vi "jigglePlatform.vi"(6 "mazeDirection":string, 9 "up or down":string, 11 "Platforms\nto jiggle":dbl[](array[numeric])) -> ()   [LabVIEW 2017]
uses:
  <vilib>/imath/engines/lvmath2/RunTimeEngine/BuiltInFunctions/length/NIMS_length(GV).vi
  <instcachedir>/0/NIMS_length(GV)_08A3D13377FD4E4B96F5795FBF3698FA.lvgen/NIMS_length(GV)_08A3D13377FD4E4B96F5795FBF3698FA_003.vi
  <vilib>/imath/engines/lvmath2/RunTimeEngine/BuiltInFunctions/repeatmx/NIMS_repeatmx(GM, I32, I32).vi
  <instcachedir>/0/NIMS_repeatmx(GM, I32, I32)_8EDBB852F26742A48D04758F158AC943.lvgen/NIMS_repeatmx(GM, I32, I32)_8EDBB852F26742A48D04758F158AC943_004.vi
  <vilib>/imath/engines/lvmath2/RunTimeEngine/RowToken/NIMS_RowToken_SorRV_M.vi
  <instcachedir>/0/NIMS_RowToken_SorRV_M_997882E9B890466D9AE38E5C4E8B9D70.lvgen/NIMS_RowToken_SorRV_M_997882E9B890466D9AE38E5C4E8B9D70_000.vi
  <vilib>/imath/engines/lvmath2/RunTimeEngine/ErrorHandling/NIMS_Create Error From Enums.vi
  <vilib>/imath/engines/lvmath2/RunTimeEngine/BuiltInFunctions/mirrorh/NIMS_mirrorh(GRowV).vi
  <instcachedir>/0/NIMS_mirrorh(GRowV)_B6A8CC4EAFBA4F9A82A59460D67BDFF0.lvgen/NIMS_mirrorh(GRowV)_B6A8CC4EAFBA4F9A82A59460D67BDFF0_000.vi
  <vilib>/imath/engines/lvmath2/RunTimeEngine/MatrixToken/NIMS_MatrixToken_RV_RV.vi
  <instcachedir>/0/NIMS_MatrixToken_RV_RV_8B087EE0EE16477EBE1C341EABB504F3.lvgen/NIMS_MatrixToken_RV_RV_8B087EE0EE16477EBE1C341EABB504F3_002.vi
  <vilib>/imathl/engines/lvmath/Functions/Error Handling/Create Error.vi
  <vilib>/imath/engines/lvmath2/RunTimeEngine/IndexRead/NIMS M($).vi
  <instcachedir>/0/NIMS M($)_82D1177398184AFB96A6AFB63C3C3F57.lvgen/NIMS M($)_82D1177398184AFB96A6AFB63C3C3F57_005.vi
  <vilib>/imath/engines/lvmath2/RunTimeEngine/MatrixToken/NIMS_MatrixToken_M_RV.vi
  <instcachedir>/0/NIMS_MatrixToken_M_RV_EE6E048DE0454E429C3E3ED099F2A9DF.lvgen/NIMS_MatrixToken_M_RV_EE6E048DE0454E429C3E3ED099F2A9DF_002.vi
  <vilib>/imath/engines/lvmath2/RunTimeEngine/NodeEndStatement/NIMS_NodeEndStatement_Output.vi
  <instcachedir>/0/NIMS_NodeEndStatement_Output_53EC0D466D134D7ABD903AC30B43404B.lvgen/NIMS_NodeEndStatement_Output_53EC0D466D134D7ABD903AC30B43404B_012.vi
  <vilib>/imath/engines/lvmath2/RunTimeEngine/ErrorHandling/NIMS_Finalize Error.vi
panel:
  out "Digital Waveform Graph 2":digitalwaveform(graph)
  out "Digital Waveform Graph 3":digitalwaveform(graph)
  out "Digital Waveform Graph":digitalwaveform(graph)
  # "Briefly move the platform.\nUsed to move platform up and down in \norder to convince animal to move."
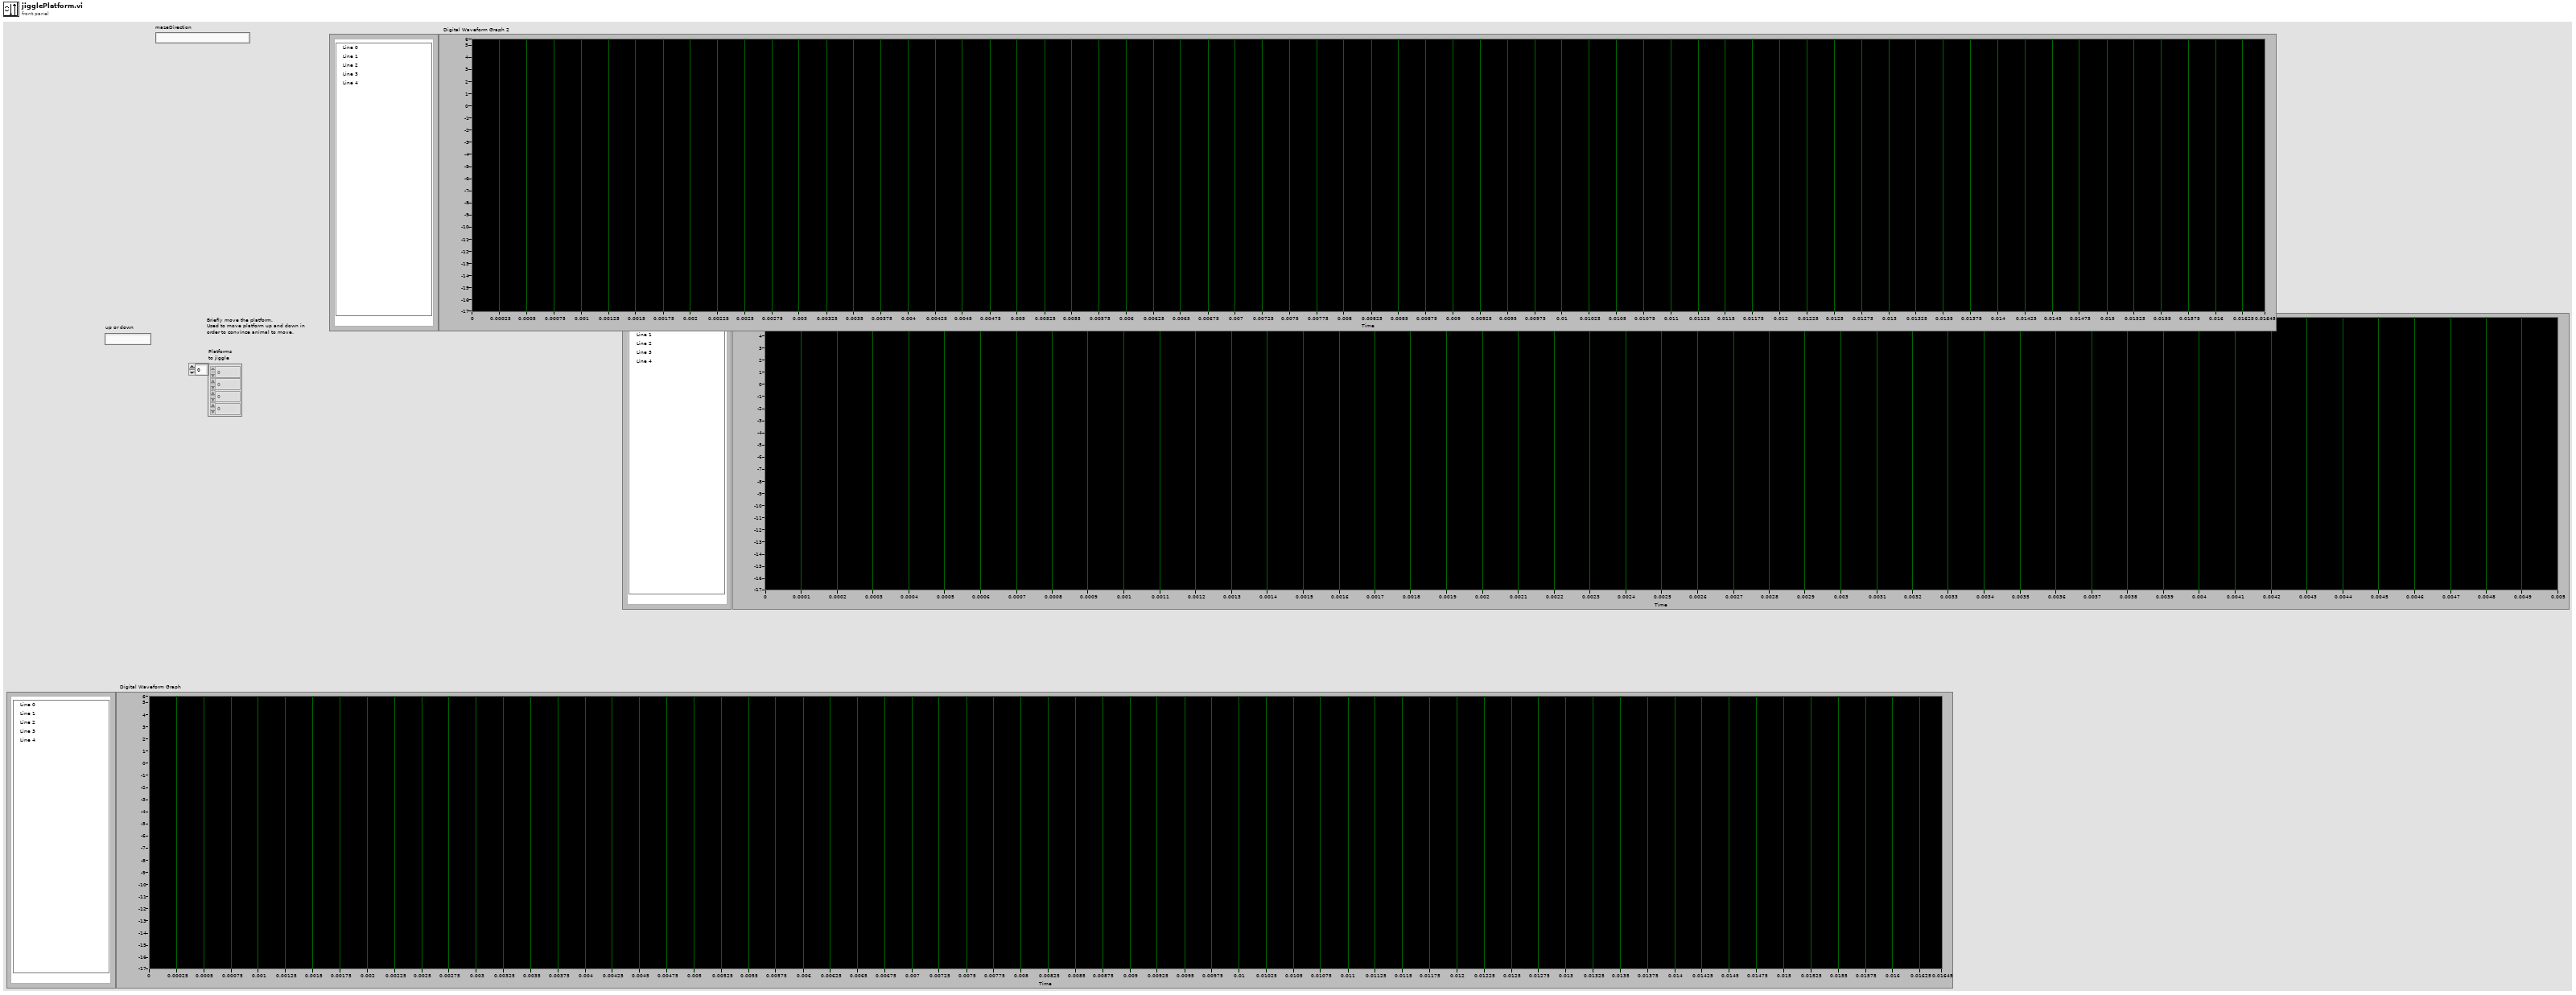
[diagram p1: front panel]
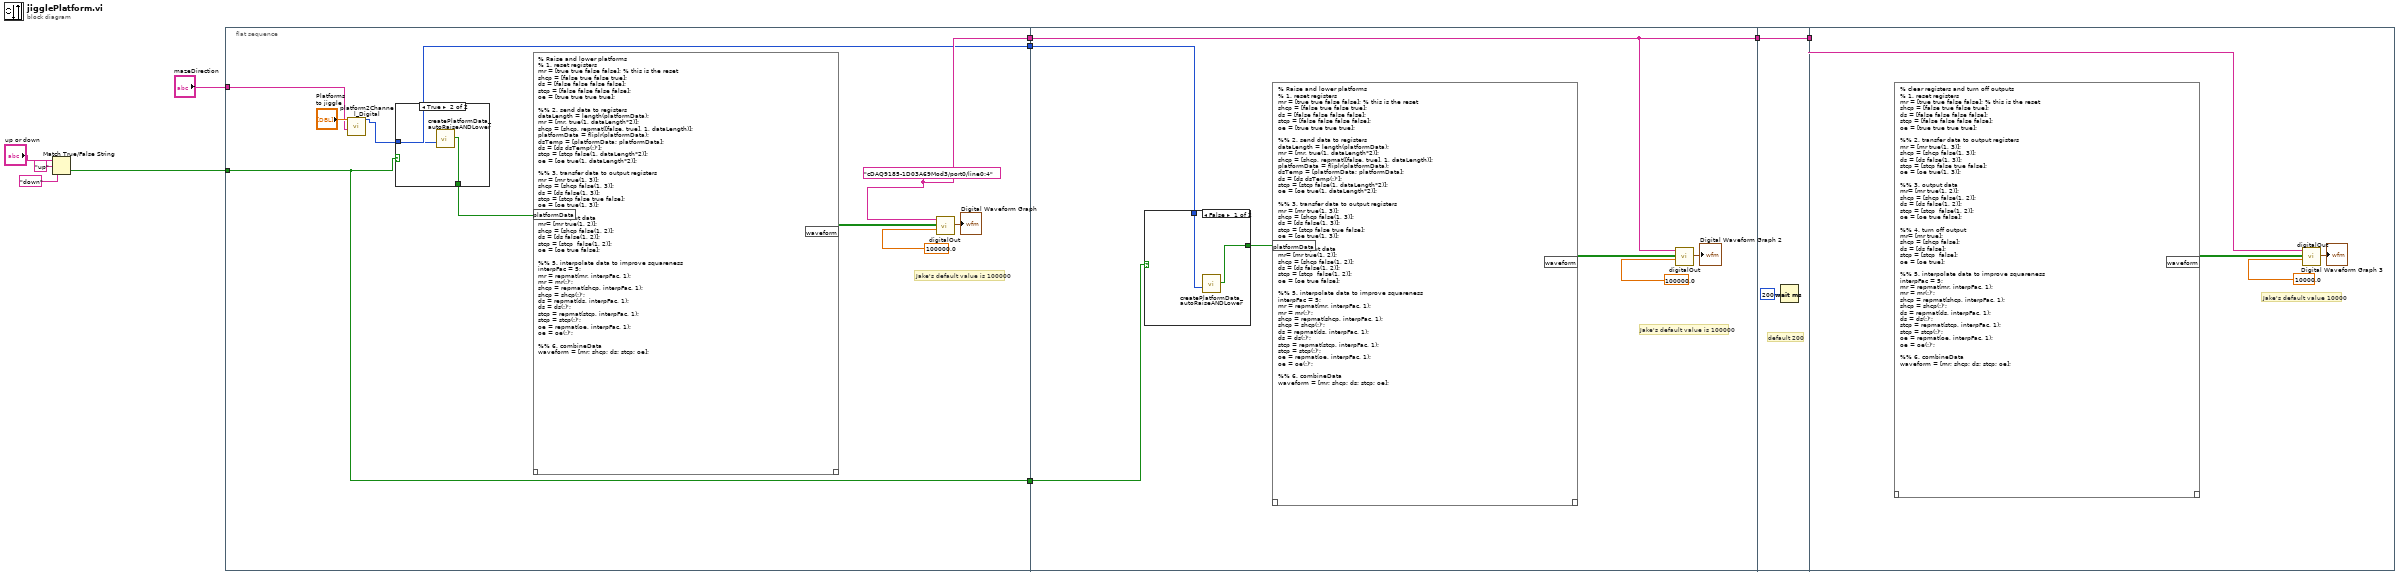
[diagram p0: block diagram]
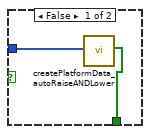
[diagram p2: hidden frame]
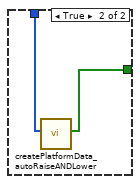
[diagram p3: hidden frame]
diagram:
  n1 = Match True/False String(2:"down" ("false string"), 3:"up" ("true string"), 4:"up or down") -> (0:w7:bool)  [unwired: 1 out]
  n2 = flat-sequence {
    tunnel: [w16] -> w4
    tunnel: [w13] -> w3
    tunnel: w7 -> [w12]
    tunnel: [w12] -> w2
    tunnel: "mazeDirection" -> [w11]
    tunnel: w4 -> [w498]
    tunnel: [w498] -> w6
    tunnel: w3 -> [w497]
    tunnel: w2 -> [w496]
    tunnel: w6 -> [w980]
    tunnel: [w980] -> w5
    tunnel: w5 -> [w981]
    frame #0 {
      w16 = tag "cDAQ9185-1D03A69Mod3/port0/line0:4" ("lines")
      # "Jake's default value is 100000"
      n3 = call "platform2Channel_Digital.vi"("mazeDirection"=w11, "Platforms"="Platforms\nto jiggle") -> ("channels"=w13:i32[])  [unwired: 9 in]
      n4 = case shown="True" w12 {
        tunnel: [w20 w23] -> w15
        tunnel: w13 -> [w21 w22]
        frame False {
          n5 = call "createPlatformData_autoRaiseANDLower.vi"("Plaforms to raise"=w21) -> ("platformData"=w20:bool[])  [unwired: 9 in]
        }
        frame True {
          n6 = call "createPlatformData_autoRaiseANDLower.vi"("Plaforms to lower"=w22) -> ("platformData"=w23:bool[])  [unwired: 9 in]
        }
      }
      n7 = mathscript code="% Raise and lower platforms\n% 1. reset registers\nmr = [true true false false]; % this is the reset\nshcp = [false true false true];\nds = [false false false false];\nstcp = [false false false false];\noe = [true true true true];\n\n%% 2. send data to registers\ndataLength = length(platformData); \nmr = [mr, true(1, dataLength*2)];\nshcp = [shcp, repmat([false, true], 1, dataLength)];\nplatformData = fliplr(platformData);\ndsTemp = [platformData; platformData];\nds = [ds dsTemp(:)'];\nstcp = [stcp false(1, dataLength*2)];\noe = [oe true(1, dataLength*2)];\n\n%% 3. transfer data to output registers\nmr = [mr true(1, 3)];\nshcp = [shcp false(1, 3)];\nds = [ds false(1, 3)];\nstcp = [stcp false true false];\noe = [oe true(1, 3)];\n\n%% 4. output data\nmr= [mr true(1, 2)];\nshcp = [shcp false(1, 2)];\nds = [ds false(1, 2)];\nstcp = [stcp  false(1, 2)];\noe = [oe true false];\n\n%% 5. interpolate data to improve squareness\ninterpFac = 5;\nmr = repmat(mr, interpFac, 1);\nmr = mr(:)';\nshcp = repmat(shcp, interpFac, 1);\nshcp = shcp(:)';\nds = repmat(ds, interpFac, 1);\nds = ds(:)';\nstcp = repmat(stcp, interpFac, 1);\nstcp = stcp(:)';\noe = repmat(oe, interpFac, 1);\noe = oe(:)';\n\n%% 6. combineData\nwaveform = [mr; shcp; ds; stcp; oe];"("platformData"=w15) -> ("waveform"=w18:bool[][])  [unwired: 1 in, 1 out]
      n8 = call "digitalOut.vi"("rate"=100000.0, "waveform"=w18, "lines"=w16) -> ("digital waveform"=→"Digital Waveform Graph":digitalwaveform)  [unwired: 8 in]
    }
    frame #1 {
      # "Jake's default value is 100000"
      n9 = case shown="False" w496 {
        tunnel: [w503 w506] -> w499
        tunnel: w497 -> [w504 w505]
        frame False {
          n10 = call "createPlatformData_autoRaiseANDLower.vi"("Plaforms to lower"=w504) -> ("platformData"=w503:bool[])  [unwired: 9 in]
        }
        frame True {
          n11 = call "createPlatformData_autoRaiseANDLower.vi"("Plaforms to raise"=w505) -> ("platformData"=w506:bool[])  [unwired: 9 in]
        }
      }
      n12 = mathscript code="% Raise and lower platforms\n% 1. reset registers\nmr = [true true false false]; % this is the reset\nshcp = [false true false true];\nds = [false false false false];\nstcp = [false false false false];\noe = [true true true true];\n\n%% 2. send data to registers\ndataLength = length(platformData); \nmr = [mr, true(1, dataLength*2)];\nshcp = [shcp, repmat([false, true], 1, dataLength)];\nplatformData = fliplr(platformData);\ndsTemp = [platformData; platformData];\nds = [ds dsTemp(:)'];\nstcp = [stcp false(1, dataLength*2)];\noe = [oe true(1, dataLength*2)];\n\n%% 3. transfer data to output registers\nmr = [mr true(1, 3)];\nshcp = [shcp false(1, 3)];\nds = [ds false(1, 3)];\nstcp = [stcp false true false];\noe = [oe true(1, 3)];\n\n%% 4. output data\nmr= [mr true(1, 2)];\nshcp = [shcp false(1, 2)];\nds = [ds false(1, 2)];\nstcp = [stcp  false(1, 2)];\noe = [oe true false];\n\n%% 5. interpolate data to improve squareness\ninterpFac = 5;\nmr = repmat(mr, interpFac, 1);\nmr = mr(:)';\nshcp = repmat(shcp, interpFac, 1);\nshcp = shcp(:)';\nds = repmat(ds, interpFac, 1);\nds = ds(:)';\nstcp = repmat(stcp, interpFac, 1);\nstcp = stcp(:)';\noe = repmat(oe, interpFac, 1);\noe = oe(:)';\n\n%% 6. combineData\nwaveform = [mr; shcp; ds; stcp; oe];"("platformData"=w499) -> ("waveform"=w501:bool[][])  [unwired: 1 in, 1 out]
      n13 = call "digitalOut.vi"("rate"=100000.0, "waveform"=w501, "lines"=w498) -> ("digital waveform"=→"Digital Waveform Graph 2":digitalwaveform)  [unwired: 8 in]
    }
    frame #2 {
      # "default 200"
      n14 = Wait (ms)(milliseconds to wait=u32 200) -> ()  [unwired: 1 out]
    }
    frame #3 {
      # "Jake's default value 10000"
      n15 = mathscript code="% clear registers and turn off outputs\n% 1. reset registers\nmr = [true true false false]; % this is the reset\nshcp = [false true false true];\nds = [false false false false];\nstcp = [false false false false];\noe = [true true true true];\n\n%% 2. transfer data to output registers\nmr = [mr true(1, 3)];\nshcp = [shcp false(1, 3)];\nds = [ds false(1, 3)];\nstcp = [stcp false true false];\noe = [oe true(1, 3)];\n\n%% 3. output data \nmr= [mr true(1, 2)];\nshcp = [shcp false(1, 2)];\nds = [ds false(1, 2)];\nstcp = [stcp  false(1, 2)];\noe = [oe true false];\n\n%% 4. turn off output\nmr= [mr true];\nshcp = [shcp false];\nds = [ds false];\nstcp = [stcp  false];\noe = [oe true];\n\n%% 5. interpolate data to improve squareness\ninterpFac = 5;\nmr = repmat(mr, interpFac, 1);\nmr = mr(:)';\nshcp = repmat(shcp, interpFac, 1);\nshcp = shcp(:)';\nds = repmat(ds, interpFac, 1);\nds = ds(:)';\nstcp = repmat(stcp, interpFac, 1);\nstcp = stcp(:)';\noe = repmat(oe, interpFac, 1);\noe = oe(:)';\n\n%% 6. combineData\nwaveform = [mr; shcp; ds; stcp; oe];"() -> ("waveform"=w983:bool[][])  [unwired: 1 in, 1 out]
      n16 = call "digitalOut.vi"("rate"=10000.0, "waveform"=w983, "lines"=w981) -> ("digital waveform"=→"Digital Waveform Graph 3":digitalwaveform)  [unwired: 8 in]
    }
  }
